vi "HandleDrive.vi"(7 "Deadzone":dbl=0.1, 8 "StraightDrive":bool, 9 "HalfDrive":bool, 10 "RightMotor":dbl, 11 "LeftMotor":dbl) -> (1 "Enqueue?":bool, 2 "RightMotor":dbl, 3 "LeftMotor":dbl)   [LabVIEW 2013]
doc: "Determines whether to enqueue a drive instruction. \nIf either joystick is outside the deadzone or half/straight drive is flipped, Enqueue? outputs true.\nIf the joysticks have just entered the deadzone, the motor outputs are set to 0 and Enqueue? outputs true.\nIf they are still in the deadzone (and previously were), Enqueue? outputs false."
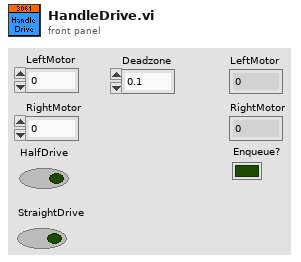
[diagram p1: front panel]
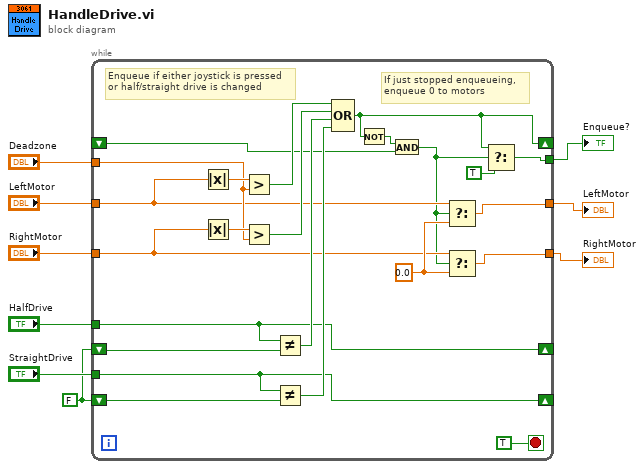
[diagram p0: block diagram]
diagram:
  w5 = FALSE ("HalfDrive")
  n1 = while {
    tunnel: "HalfDrive" -> [w27]
    tunnel: "LeftMotor" -> [w18]
    tunnel: "RightMotor" -> [w19]
    tunnel: "StraightDrive" -> [w26]
    shift-right: [w27] -> _
    shift-left: w5 -> [w28]
    shift-right: [w26] -> _
    shift-left: w5 -> [w29]
    tunnel: "Deadzone" -> [w23]
    tunnel: [w17] -> w3
    tunnel: [w16] -> w2
    shift-right: [w11] -> _
    shift-left: _ -> [w12]
    tunnel: [w15] -> w1
    stop <- TRUE stop-if-true
    w20 = 0.0
    # "Enqueue if either joystick is pressed\nor half/straight drive is changed"
    # "If just stopped enqueueing,\nenqueue 0 to motors"
    n2 = Absolute Value(x=w18) -> (abs(x)=w24:dbl)
    n3 = Absolute Value(x=w19) -> (abs(x)=w25:dbl)
    n4 = Greater?(x=w24, y=w23) -> (0:w22:bool)
    n5 = Greater?(x=w25, y=w23) -> (0:w21:bool)
    n6 = Not Equal?(x=w27, y=w28) -> (x != y?=w30:bool)
    n7 = Not Equal?(x=w26, y=w29) -> (x != y?=w31:bool)
    n8 = Compound Arithmetic op=OR(w22, w21, w30, w31) -> (w11:bool)
    n9 = Not(x=w11) -> (.not. x?=w10:bool)
    n10 = And(x=w10, y=w12) -> (x .and. y?=w13:bool)
    n11 = Select(t=w18, s=w13, f=w20) -> (s? t:f=w17:dbl)
    n12 = Select(t=w19, s=w13, f=w20) -> (s? t:f=w16:dbl)
    n13 = Select(t=w11, s=w13, f=TRUE) -> (s? t:f=w15:bool)
  }
  "Enqueue?" <- w1
  "RightMotor" <- w2
  "LeftMotor" <- w3
